vi "Set Bucket Website Configuration.vi"(4 "Region":T1, 7 "WebsiteConfiguration":T2, 8 "error in (no error)":errorcluster, 9 "Bucket":string) -> (0 "error out":errorcluster)   [LabVIEW 2015, in "LV Interface for Amazon S3.lvlib"]
doc: "This operation <B>sets the website configuration</B>. This operation <B>requires the S3:PutBucketWebsite permission</B>. By default, <B>only the bucket owner can configure the website attached to a bucket</B>. However, bucket <B>owners can allow other users to set the website configuration by</B> writing a bucket policy <B>granting them the S3:PutBucketWebsite permission</B>.\n\n<b>Note:</b> If the <b>RedirectAllRequestsTo</b> value is specified, all other values in the <b>WebsiteConfiguration</b> are ignored. If the <b>RedirectAllRequestsTo</b> value is an empty string, then the remaining values are used to set the bucket website configuration."
uses:
  LV Interface for Amazon S3.lvlib
  Typedefs/AMZ_S3_API_WebsiteConfiguration.ctl
  Typedefs/AMZ_S3_LocationConstraint.ctl
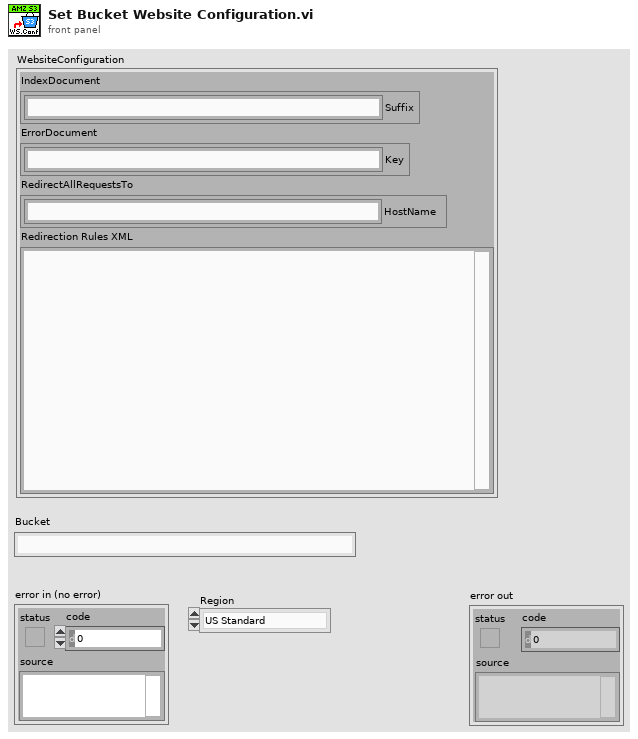
[diagram p1: front panel]
types:
  T1 = typedef "LV Interface for Amazon S3.lvlib/AMZ_S3_LocationConstraint.ctl" = enum16{"US Standard", "us-east-2", "us-west-1", "us-west-2", "ap-northeast-1", "ap-northeast-2", "ap-southeast-1", "ap-southeast-2", "ca-central-1", "eu-central-1", "eu-west-1", "eu-west-2", "sa-east-1"}
  T2 = typedef "LV Interface for Amazon S3.lvlib/AMZ_S3_API_WebsiteConfiguration.ctl" = cluster{"IndexDocument":cluster{"Suffix":string}, "ErrorDocument":cluster{"Key":string}, "RedirectAllRequestsTo":cluster{"HostName":string}, "Redirection Rules XML":string}
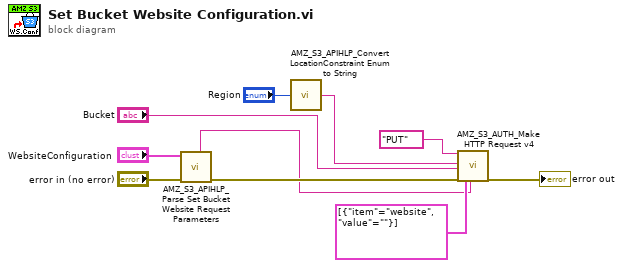
[diagram p0: block diagram]
diagram:
  n1 = call "AMZ_S3_APIHLP_Parse Set Bucket Website Request Parameters.vi"("error in (no error)"="error in (no error)", "Website Configuration"="WebsiteConfiguration") -> ("error out"=w6:errorcluster, "PUT Data"=w4:string)  [unwired: 8 in]
  n2 = call "AMZ_S3_APIHLP_Convert LocationConstraint Enum to String.vi"("Location"="Region") -> ("Location String"=w2:string)  [unwired: 4 in]
  n3 = call "AMZ_S3_AUTH_Make HTTP Request v4.vi"("HTTP-Verb"="PUT", "Region"=w2, "Bucket"="Bucket", "error in"=w6, "request parameters"=cluster{"item":string, "value":string}[] [{"item"="website", "value"=""}], "request body"=w4) -> ("error out"=→"error out":errorcluster)  [unwired: 10 in, 3 out]
